vi "Dynamic Load Ruby.vi"(8 "Error In":errorcluster) -> (0 "Error Out":errorcluster, 2 "Device names":string[](array[string]), 3 "Digitizers out":refnum<class "Instrument Actor.lvclass">[](array[class]))   [LabVIEW 2018]
uses:
  Instrument Actor/Instrument Actor.lvclass
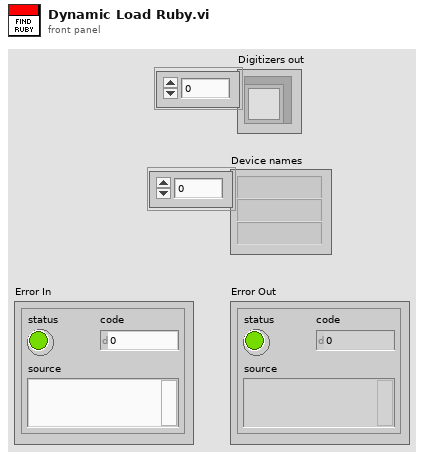
[diagram p1: front panel]
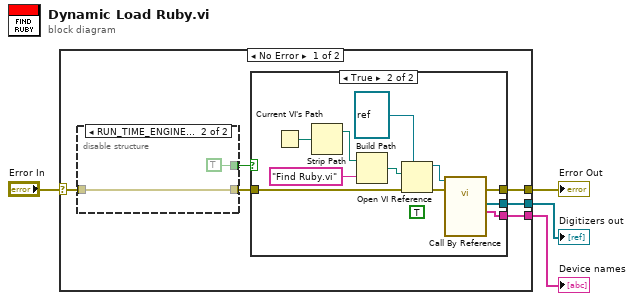
[diagram p0: block diagram]
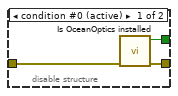
[diagram p2: hidden frame]
diagram:
  n1 = case shown="No Error" "Error In" {
    selector: "Error In" -> [w8 w28]
    tunnel: [w10 w28] -> w2
    tunnel: [w6 _] -> w4
    tunnel: [w5 _] -> w3
    frame No Error {
      n2 = disable-structure shown="RUN_TIME_ENGINE==True" {
        disable-tunnel: [w13 TRUE ("file or folder exists?")] -> w9
        disable-tunnel: w8 -> [w12 w15]
        disable-tunnel: [w11 w15] -> w7
        frame condition #0 (active) {
          n3 = call "Is OceanOptics installed.vi"("Error In"=w12) -> ("Error Out"=w11:errorcluster, "file or folder exists?"=w13:bool)  [unwired: 9 in]
        }
        frame condition #1 {
        }
      }
      n4 = case shown="True" w9 {
        tunnel: w7 -> [w16 w22]
        tunnel: [w16 w19] -> w10
        tunnel: [_ w20] -> w6
        tunnel: [_ w17] -> w5
        frame False {
        }
        frame True {
          (unwired) TRUE ("DAQmx loaded")
          n5 = Current VI's Path() -> (path=w26:path)
          n6 = Strip Path(path=w26) -> (stripped path=w18:path)  [unwired: 1 out]
          n7 = Build Path(base path=w18, name or relative path="Find Ruby.vi") -> (appended path=w21:path)
          n8 = Open VI Reference(type specifier VI Refnum (for type only)=refnum<vi> refnum, vi path=w21, error in (no error)=w22) -> (vi reference=w24:refnum<vi>, error out=w23:errorcluster)  [unwired: 3 in]
          n9 = call-by-ref "?"(reference=w24, error in=w23) -> (error out=w19:errorcluster, "Names"=w20:string[], "Recorders List"=w17:refnum<class "Instrument Actor.lvclass">[])  [unwired: 9 in, 2 out]
        }
      }
    }
    frame Error {
    }
  }
  "Error Out" <- w2
  "Digitizers out" <- w3
  "Device names" <- w4
